vi "R0NetworkHealthCheck.vi"() -> (2 "Percentage Write Success":dbl, 3 "CPU loads":T1[](array[typedef]) {"ISR (%)" format="%#.2f"; "Idle (%)" format="%#.2f"; "Background (%)" format="%#.2f"; "Normal (%)" format="%#.2f"; "Above Normal (%)" format="%#.2f"; "High (%)" format="%#.2g"; "Timed Structures (%)" format="%#.2g"; "Time Critical (%)" format="%#.2g"; "Total (%)" format="%#.2g"})   [LabVIEW 2016]
uses:
  <vilib>/Utility/RT CPU Load.ctl
  <vilib>/wsapi/Web Request.lvclass
  <vilib>/Analysis/baseanly.llb/Mean (DBL).vi
  <vilib>/NI_Real-Time Target Support.lvlib
  <vilib>/Analysis/NI_AALBase.lvlib
panel:
  in  "LabVIEW Web Service Request":refnum<class "Web Request.lvclass">
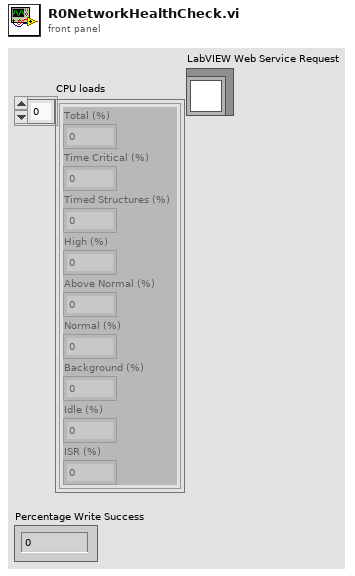
[diagram p1: front panel]
types:
  T1 = typedef "NI_Real-Time Target Support.lvlib/RT CPU Load.ctl" = cluster{"Total (%)":dbl, "Time Critical (%)":dbl, "Timed Structures (%)":dbl, "High (%)":dbl, "Above Normal (%)":dbl, "Normal (%)":dbl, "Background (%)":dbl, "Idle (%)":dbl, "ISR (%)":dbl}
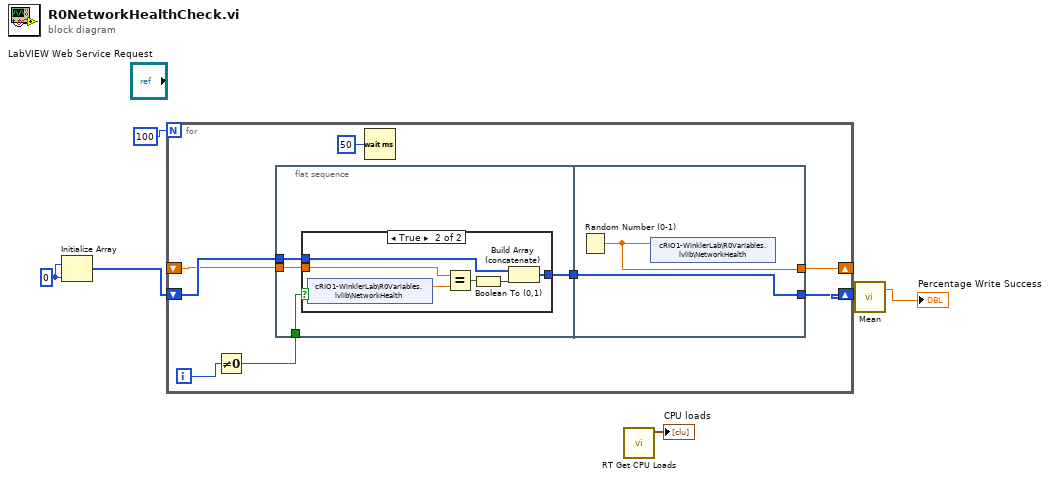
[diagram p0: block diagram]
diagram:
  w1 = 0 ("dimension size")
  n1 = Initialize Array(w1, w1) -> (w2:i32[])
  n2 = for {
    N: 100 -> [_]
    shift-right: [w10] -> w4
    shift-left: w2 -> [w14]
    shift-right: [w12] -> _
    shift-left: _ -> [w13]
    i -> [w7]
    n3 = Not Equal To 0?(x=w7) -> (x != 0?=w8:bool)
    n4 = flat-sequence {
      tunnel: w13 -> [w18]
      tunnel: w14 -> [w16]
      tunnel: [w17] -> w9
      tunnel: w8 -> [w15]
      tunnel: [w27] -> w12
      tunnel: [w26] -> w10
      tunnel: w9 -> [w26]
      frame #0 {
        n5 = case shown="True" w15 {
          tunnel: w18 -> [_ w24]
          tunnel: [w19 w21] -> w17
          tunnel: w16 -> [w19 w20]
          frame False {
          }
          frame True {
            n6 = shared-variable "cRIO1-WinklerLab\\R0Variables.lvlib\\NetworkHealth"() -> (w25:dbl)  [unwired: 1 in, 1 out]
            n7 = Equal?(x=w24, y=w25) -> (x = y?=w23:bool)
            n8 = Boolean To (0,1)(Boolean=w23) -> (0, 1=w22:i16)
            n9 = Build Array (concatenate)(w20, w22) -> (w21:i32[])
          }
        }
      }
      frame #1 {
        n10 = Random Number (0-1)() -> (number: 0 to 1=w27:dbl)
        n11 = shared-variable "cRIO1-WinklerLab\\R0Variables.lvlib\\NetworkHealth"(w27) -> ()  [unwired: 1 in, 1 out]
      }
    }
    n12 = Wait (ms)(milliseconds to wait=u32 50) -> ()  [unwired: 1 out]
  }
  n13 = call <vilib>:"RT Get CPU Loads.vi"() -> ("CPU loads"=→"CPU loads":T1[])  [unwired: 10 in, 1 out]
  n14 = call-poly <vilib>:"Mean.vi"("X"=w4) -> ("mean"=→"Percentage Write Success":dbl)  [unwired: 1 out]
